vi "target.vi"() -> ()   [LabVIEW 2020]
uses:
  <vilib>/Platform/TimedLoop/XDataNode/timing_clust.ctl
  <vilib>/Platform/TimedLoop/XDataNode/nitl_modes.ctl
  <vilib>/Platform/TimedLoop/XDataNode/wakeup.ctl
  <vilib>/Analysis/Matrix/Numeric/Conversions/Array To Matrix - RA.vi
  <vilib>/Platform/TimedLoop/XDataNode/loadnilvce.vi
  <vilib>/Analysis/Matrix/Numeric/Conversions/Array To Matrix - RA2.vi
  <vilib>/Analysis/Matrix/Numeric/Conversions/Matrix To Array - RM.vi
  <vilib>/platform/TimedLoop/XDataNode/XDataNode.xnode
  <vilib>/Platform/TimedLoop/XDataNode/XDNodeRunTimeDep.lvlib
  <vilib>/Analysis/Matrix/NI_Matrix.lvlib
panel:
  out "Waveform Chart":dbl(graph)
  in  "stop":bool
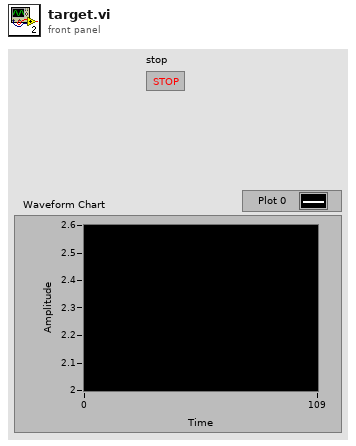
[diagram p1: front panel]
types:
  T1 = typedef "NI_Matrix.lvlib/RealMatrix.ctl" = dbl[][]
  T2 = typedef "XDNodeRunTimeDep.lvlib/timing_clust.ctl" = cluster{"Expected End [f-1]":u64, "Actual End [f-1]":u64, "Finished Late? [f-1]":bool, "Expected End [i-1]":u64, "Actual End [i-1]":u64, "Finished Late? [i-1]":bool, "Expected Start [i]":u64, "Actual Start [i]":u64, "Expected Start [f]":u64, "Actual Start [f]":u64, "Source Name":string, "Structure Name":string, "Period":i64, "Deadline":i64, "Offset":i64, "Start":i64, "Priority":i32, "Timeout":i32, "Mode":T3, "Wakeup Reason":T4, "Error":errorcluster, "Source Type":string, "Secondary Source Type":string, "Global End Time":u64, "Global Start Time":u64, "Frame Duration":u64, "Iteration Duration":u64, "Assigned CPU":i32, "I/O Scan Engine Mode":u32}
  T3 = typedef "XDNodeRunTimeDep.lvlib/nitl_modes.ctl" = enum32{"No Change", "Process missed periods, maintain original phase", "Discard missed periods, maintain original phase", "Process missed periods, ignore original phase", "Discard missed periods, ignore original phase"}
  T4 = typedef "XDNodeRunTimeDep.lvlib/wakeup.ctl" = enum32{"Normal", "Aborted", "Asynchronous wakeup", "Timing source error", "Timed loop error", "Timeout"}
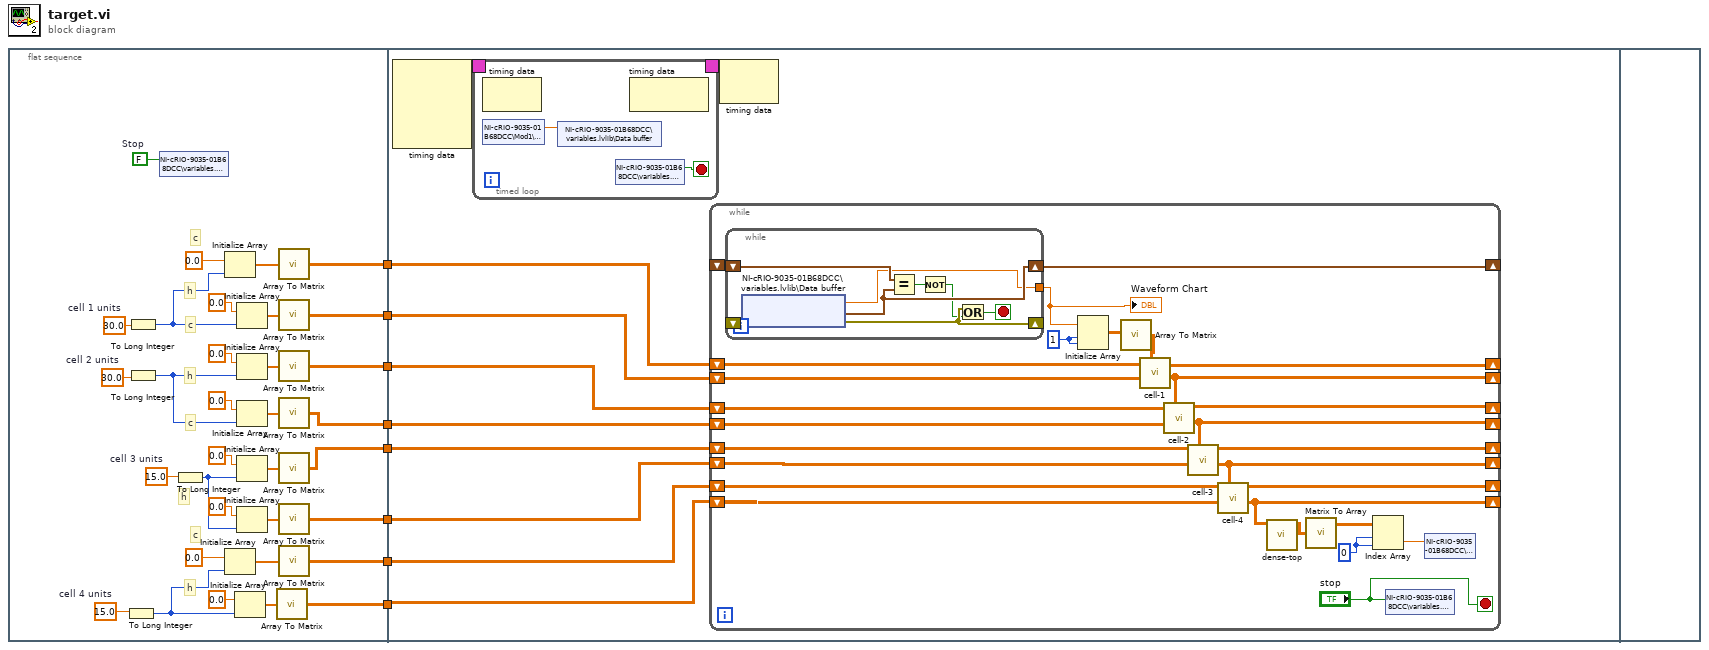
[diagram p0: block diagram]
diagram:
  n1 = flat-sequence {
    tunnel: [w17] -> w8
    tunnel: [w16] -> w7
    tunnel: [w15] -> w6
    tunnel: [w14] -> w5
    tunnel: [w13] -> w4
    tunnel: [w12] -> w3
    tunnel: [w11] -> w2
    tunnel: [w10] -> w1
    tunnel: w8 -> [w49]
    tunnel: w7 -> [w48]
    tunnel: w6 -> [w47]
    tunnel: w5 -> [w46]
    tunnel: w4 -> [w45]
    tunnel: w3 -> [w44]
    tunnel: w2 -> [w43]
    tunnel: w1 -> [w42]
    frame #0 {
      w9 = FALSE  # Stop
      w25 = 15.0  # cell 4 units
      w23 = 15.0  # cell 3 units
      w21 = 30.0  # cell 2 units
      w19 = 30.0  # cell 1 units
      # "c"
      # "c"
      # "c"
      # "c"
      # "h"
      # "h"
      # "h"
      # "h"
      n2 = To Long Integer(number=w25) -> (32bit integer=w41:i32)
      n3 = To Long Integer(number=w19) -> (32bit integer=w35:i32)
      n4 = To Long Integer(number=w21) -> (32bit integer=w37:i32)
      n5 = shared-variable "NI-cRIO-9035-01B68DCC\\variables.lvlib\\Stop"(w9) -> ()  [unwired: 1 in, 1 out]
      n6 = To Long Integer(number=w23) -> (32bit integer=w39:i32)
      n7 = Initialize Array(0.0, w35) -> (w34:dbl[])
      n8 = Initialize Array(0.0, w41) -> (w40:dbl[])
      n9 = Initialize Array(0.0, w41) -> (w33:dbl[])
      n10 = Initialize Array(0.0, w35) -> (w30:dbl[])
      n11 = Initialize Array(0.0, w37) -> (w36:dbl[])
      n12 = Initialize Array(0.0, w37) -> (w31:dbl[])
      n13 = Initialize Array(0.0, w39) -> (w38:dbl[])
      n14 = Initialize Array(0.0, w39) -> (w32:dbl[])
      n15 = call-poly <vilib>:"Array To Matrix.vi"("Real 1D Array"=w33) -> ("Real Matrix (Column Vector)"=w10:T1)
      n16 = call-poly <vilib>:"Array To Matrix.vi"("Real 1D Array"=w34) -> ("Real Matrix (Column Vector)"=w17:T1)
      n17 = call-poly <vilib>:"Array To Matrix.vi"("Real 1D Array"=w30) -> ("Real Matrix (Column Vector)"=w16:T1)
      n18 = call-poly <vilib>:"Array To Matrix.vi"("Real 1D Array"=w36) -> ("Real Matrix (Column Vector)"=w15:T1)
      n19 = call-poly <vilib>:"Array To Matrix.vi"("Real 1D Array"=w31) -> ("Real Matrix (Column Vector)"=w14:T1)
      n20 = call-poly <vilib>:"Array To Matrix.vi"("Real 1D Array"=w38) -> ("Real Matrix (Column Vector)"=w13:T1)
      n21 = call-poly <vilib>:"Array To Matrix.vi"("Real 1D Array"=w32) -> ("Real Matrix (Column Vector)"=w12:T1)
      n22 = call-poly <vilib>:"Array To Matrix.vi"("Real 1D Array"=w40) -> ("Real Matrix (Column Vector)"=w11:T1)
    }
    frame #1 {
      n23 = node-c288() -> (w51:T2)  [unwired: 4 in]
      n24 = timed-loop {
        timing: w51 -> [_]
        timing-out: [_] -> w50
        stop <- w87 stop-if-true
        n25 = node-c288() -> ()  [unwired: 1 in, 1 out]
        n26 = shared-variable "NI-cRIO-9035-01B68DCC\\Mod1\\AI0"() -> (w88:dbl)  [unwired: 1 in, 1 out]
        n27 = shared-variable "NI-cRIO-9035-01B68DCC\\variables.lvlib\\Data buffer"(w88) -> ()  [unwired: 1 in, 1 out]
        n28 = shared-variable "NI-cRIO-9035-01B68DCC\\variables.lvlib\\Stop"() -> (w87:bool)  [unwired: 1 in, 1 out]
        n29 = node-c288() -> ()  [unwired: 1 in, 1 out]
      }
      n30 = while {
        shift-right: [w66] -> _
        shift-left: w49 -> [w78]
        shift-right: [w67] -> _
        shift-left: w48 -> [w77]
        shift-right: [w64] -> _
        shift-left: w47 -> [w76]
        shift-right: [w65] -> _
        shift-left: w46 -> [w75]
        shift-right: [w62] -> _
        shift-left: w45 -> [w74]
        shift-right: [w63] -> _
        shift-left: w44 -> [w73]
        shift-right: [w61] -> _
        shift-left: w43 -> [w72]
        shift-right: [w58] -> _
        shift-left: w42 -> [w71]
        shift-right: [w70] -> _
        shift-left: _ -> [w69]
        stop <- "stop" stop-if-true
        w56 = 0
        w68 = 1
        n31 = while {
          shift-right: [w85] -> w70
          shift-left: w69 -> [w84]
          shift-right: [w83] -> _
          shift-left: _ -> [w86]
          tunnel: [w79] -> w52
          stop <- w81 stop-if-true
          n32 = shared-variable "NI-cRIO-9035-01B68DCC\\variables.lvlib\\Data buffer"(error in=w86) -> (w79:dbl, error out=w83:errorcluster, w85:timestamp)
          n33 = Equal?(x=w84, y=w85) -> (x = y?=w80:bool)
          n34 = Not(x=w80) -> (.not. x?=w82:bool)
          n35 = Or(x=w83, y=w82) -> (x .or. y?=w81:bool)
        }
        "Waveform Chart" <- w52
        n36 = Initialize Array(w52, w68, w68) -> (w60:dbl[][])
        n37 = call-poly <vilib>:"Array To Matrix.vi"("Real 2D Array"=w60) -> ("Real Matrix"=w59:T1)
        n38 = call "cell-1.vi"("x"=w59, "h"=w77, "c"=w78) -> ("h + 1"=w67:T1, "c + 1"=w66:T1)  [unwired: 7 in]
        n39 = call "cell-2.vi"("x"=w67, "h"=w75, "c"=w76) -> ("h + 1"=w65:T1, "c + 1"=w64:T1)  [unwired: 7 in]
        n40 = call "cell-3.vi"("x"=w65, "h"=w73, "c"=w74) -> ("h + 1"=w63:T1, "c + 1"=w62:T1)  [unwired: 7 in]
        n41 = call "cell-4.vi"("x"=w63, "h"=w71, "c"=w72) -> ("h + 1"=w58:T1, "c + 1"=w61:T1)  [unwired: 7 in]
        n42 = call "dense-top.vi"("x_dense"=w58) -> ("y_out"=w55:T1)  [unwired: 10 in]
        n43 = call-poly <vilib>:"Matrix To Array.vi"("Real Matrix"=w55) -> ("Real 2D Array"=w57:dbl[][])
        n44 = Index Array(array=w57, index (row)=w56, index (col)=w56) -> (element=w53:dbl)
        n45 = shared-variable "NI-cRIO-9035-01B68DCC\\variables.lvlib\\Stop"("stop") -> ()  [unwired: 1 in, 1 out]
        n46 = shared-variable "NI-cRIO-9035-01B68DCC\\variables.lvlib\\y"(w53) -> ()  [unwired: 1 in, 1 out]
      }
      n47 = node-c288(w50) -> ()  [unwired: 1 out]
    }
    frame #2 {
    }
  }
